vi "Set 1D Array Double.vi"(5 "use temporary file? (F)":bool, 7 "column vector?":bool, 8 "error in":errorcluster, 9 "value":dbl[](array[numeric]), 10 "variable name":string, 11 "GOLPI ref. in":T1={"pipe handle"={"lv_proc.dll file path"=path "", "process instance handle"=[], "debug mode"=FALSE, "debug data"=[]}, "fast read timeout [ms]"=500, "fast read settle time [ms]"=10, "fast read to multiple [ms]"=1, "max elements per input line"=100, "slow read timeout [ms]"=5000, "stdin double format specifier"="%_16e", "max elements per stdout output column"=100, "console mode bitstream"=FALSE, "bitstream first read timeout [ms]"=1000, "bitstream read timeout [ms]"=50, "struct transfer possible"=FALSE, "matlab mode"=FALSE, "var pipe write timeout [ms]"=5000, "variable pipe mode"=FALSE, "variable pipe buffer size [Bytes]"=10000000, "variable pipe block size [Bytes]"=1000000} {"variable pipe block size [Bytes]" format="%.0p"; "variable pipe buffer size [Bytes]" format="%.0p"}) -> (0 "error out":errorcluster, 3 "GOLPI ref. out":T1={"pipe handle"={"lv_proc.dll file path"=path "", "process instance handle"=[], "debug mode"=FALSE, "debug data"=[]}, "fast read timeout [ms]"=500, "fast read settle time [ms]"=10, "fast read to multiple [ms]"=1, "max elements per input line"=100, "slow read timeout [ms]"=5000, "stdin double format specifier"="%_16e", "max elements per stdout output column"=100, "console mode bitstream"=FALSE, "bitstream first read timeout [ms]"=1000, "bitstream read timeout [ms]"=50, "struct transfer possible"=FALSE, "matlab mode"=FALSE, "var pipe write timeout [ms]"=5000, "variable pipe mode"=FALSE, "variable pipe buffer size [Bytes]"=10000000, "variable pipe block size [Bytes]"=1000000} {"variable pipe block size [Bytes]" format="%.0p"; "variable pipe buffer size [Bytes]" format="%.0p"})   [LabVIEW 2020, in "GOLPI library.lvlib"]
doc: "Part of polymorph Set Variable.vi"
uses:
  GOLPI library.lvlib
  Public/GOLPI reference Type Def.ctl
  LV Process source distribution/Pipe Handle.ctl
  LV Process source distribution/LV Process library.lvlib
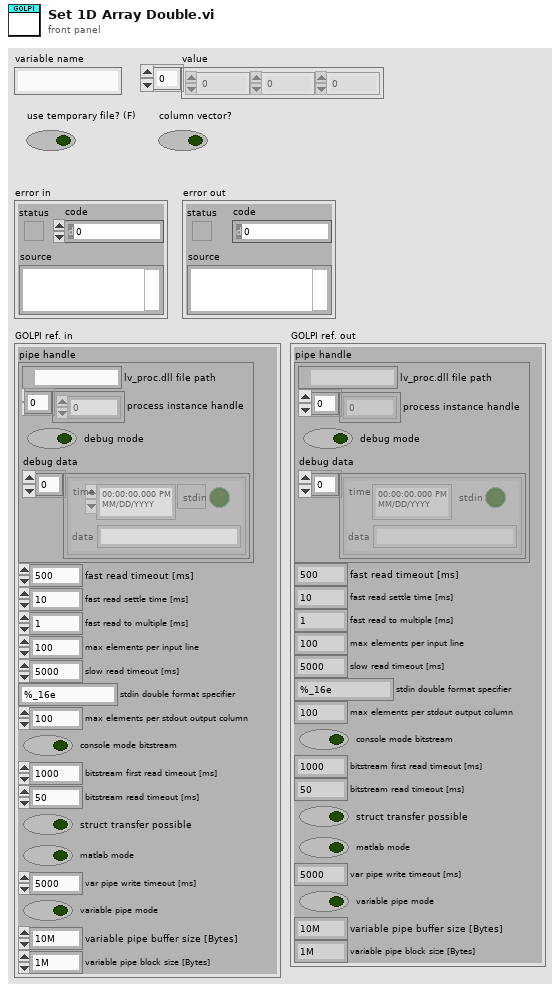
[diagram p1: front panel]
types:
  T1 = typedef "GOLPI library.lvlib/GOLPI reference Type Def.ctl" = cluster{"pipe handle":T2, "fast read timeout [ms]":u32, "fast read settle time [ms]":u32, "fast read to multiple [ms]":u32, "max elements per input line":u32, "slow read timeout [ms]":u32, "stdin double format specifier":string, "max elements per stdout output column":u32, "console mode bitstream":bool, "bitstream first read timeout [ms]":u32, "bitstream read timeout [ms]":u32, "struct transfer possible":bool, "matlab mode":bool, "var pipe write timeout [ms]":u32, "variable pipe mode":bool, "variable pipe buffer size [Bytes]":u32, "variable pipe block size [Bytes]":u32}
  T2 = typedef "LV Process library.lvlib/Pipe Handle.ctl" = cluster{"lv_proc.dll file path":path, "process instance handle":u32[], "debug mode":bool, "debug data":cluster{"time":timestamp, "stdin":bool, "data":string}[]}
  T3 = typedef "GOLPI library.lvlib/Transfer Mode.ctl" = enum16{"Matlab", "stdio", "temp file", "bitstream", "pipe"}
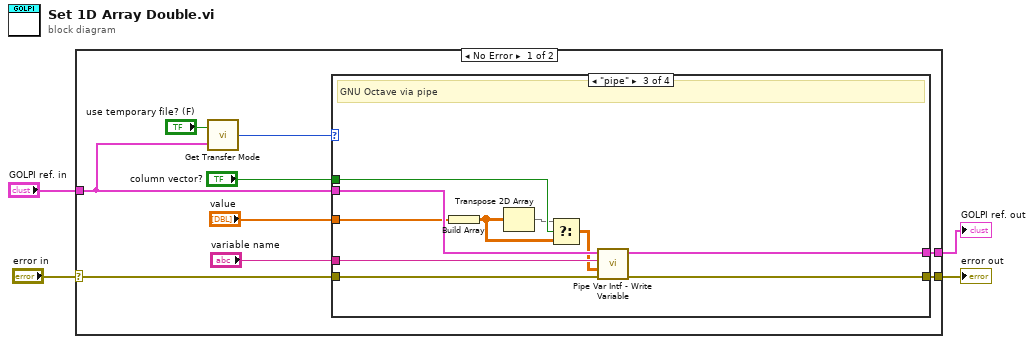
[diagram p0: block diagram]
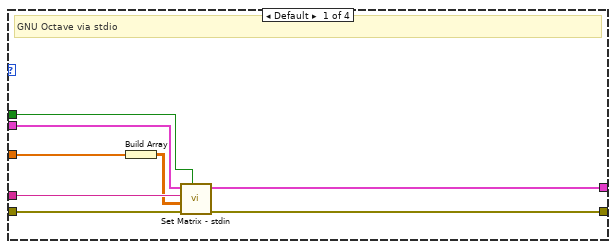
[diagram p2: hidden frame]
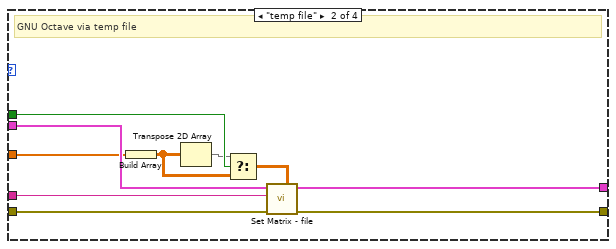
[diagram p3: hidden frame]
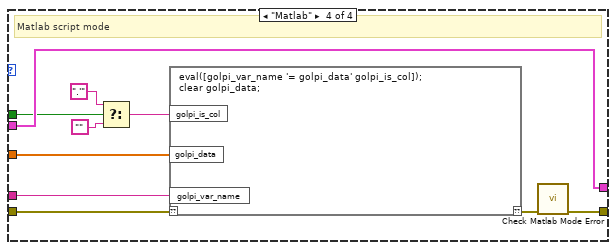
[diagram p4: hidden frame]
diagram:
  n1 = case shown="No Error" "error in" {
    selector: "error in" -> [w12 w53]
    tunnel: [w11 w53] -> w4
    tunnel: "GOLPI ref. in" -> [w7 w52]
    tunnel: [w10 w52] -> w1
    frame No Error {
      n2 = call "Get Transfer Mode.vi"("GOLPI ref."=w7, "use temporary file? (F)"="use temporary file? (F)") -> ("mode"=w5:T3)
      n3 = case shown="\"pipe\"" w5 {
        tunnel: "variable name" -> [w21 w31 w41 w50]
        tunnel: w12 -> [w20 w30 w40 w51]
        tunnel: [w19 w29 w39 w42] -> w11
        tunnel: w7 -> [w18 w28 w38 w48]
        tunnel: [w17 w27 w37 w48] -> w10
        tunnel: "value" -> [w16 w26 w36 w49]
        tunnel: "column vector?" -> [w15 w25 w35 w47]
        frame Default {
          # "GNU Octave via stdio"
          n4 = Build Array(w16) -> (w14:dbl[][])
          n5 = call "Set Matrix - stdin.vi"("swap dimensions? (F)"=w15, "error in"=w20, "value"=w14, "variable name"=w21, "GOLPI ref. in"=w18) -> ("error out"=w19:errorcluster, "GOLPI ref. out"=w17:T1)  [unwired: 5 in]
        }
        frame "temp file" {
          # "GNU Octave via temp file"
          n6 = Build Array(w26) -> (w24:dbl[][])
          n7 = Transpose 2D Array(2D array=w24) -> (transposed array=w23:dbl[][])
          n8 = Select(t=w23, s=w25, f=w24) -> (s? t:f=w22:dbl[][])
          n9 = call "Set Matrix - file.vi"("double array"=w22, "error in (no error)"=w30, "variable name"=w31, "GOLPI ref. in"=w28) -> ("error out"=w29:errorcluster, "GOLPI ref. out"=w27:T1)  [unwired: 6 in]
        }
        frame "pipe" {
          # "GNU Octave via pipe"
          n10 = Build Array(w36) -> (w34:dbl[][])
          n11 = Transpose 2D Array(2D array=w34) -> (transposed array=w33:dbl[][])
          n12 = Select(t=w33, s=w35, f=w34) -> (s? t:f=w32:dbl[][])
          n13 = call "Pipe Var Intf - Write Variable.vi"("error in (no error)"=w40, "data in"=w32, "variable name"=w41, "GOLPI ref. in"=w38) -> ("error out"=w39:errorcluster, "GOLPI ref. out"=w37:T1)  [unwired: 6 in]
        }
        frame "Matlab" {
          # "Matlab script mode"
          n14 = Select(t=".'", s=w47, f="") -> (s? t:f=w46:string)
          n15 = script code="eval([golpi_var_name '= golpi_data' golpi_is_col]);\nclear golpi_data;"("??"=w51, "golpi_var_name"=w50, "golpi_data"=w49, "golpi_is_col"=w46) -> ("??"=w43:errorcluster)
          n16 = call "Check Matlab Mode Error.vi"("error in"=w43) -> ("error out"=w42:errorcluster)  [unwired: 10 in]
        }
      }
    }
    frame Error {
    }
  }
  "error out" <- w4
  "GOLPI ref. out" <- w1
